vi "Ocean Optics 2000 4000 Acquire Continuous Waveform.vi"() -> ()   [LabVIEW 2024]
doc: "Demonstrates continuous waveform measurement. Spectrum is displayed in a waveform graph."
uses:
  Ocean Optics 2000 4000.lvlib
panel:
  in  "Stop":bool
  out "Spectral Waveform":cluster{dbl[], dbl[]}(graph)
  in  "Enable Strobe (Disabled)":bool
  in  "VISA resource name":refnum<visa-resource-name>
  # "(c) 2009-2016 National Instruments.  ALL RIGHTS RESERVED."
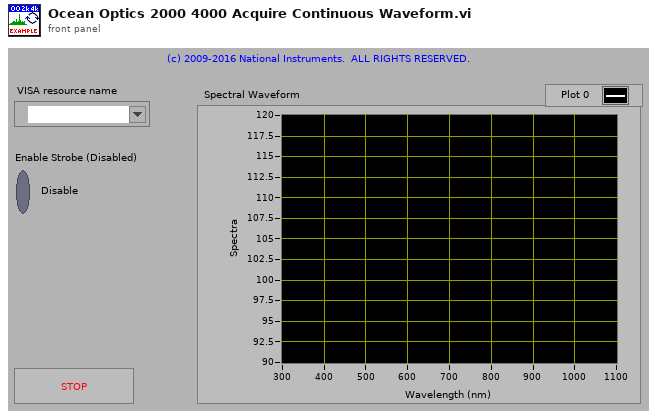
[diagram p1: front panel]
types:
  T1 = cluster{"Wavelength (nm)":dbl[], "Spectrum by Pixel Number":dbl[]}
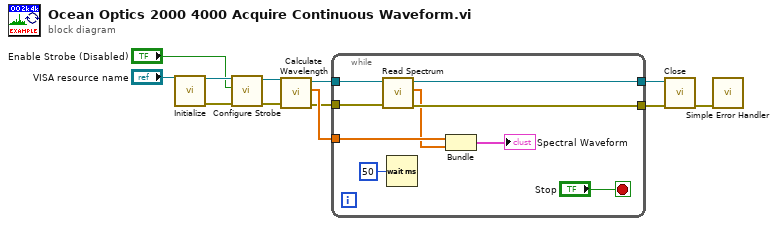
[diagram p0: block diagram]
diagram:
  n1 = call "Initialize.vi"("VISA resource name"="VISA resource name") -> ("error out"=w11:errorcluster, "VISA resource name out"=w12:refnum<visa-resource-name>)  [unwired: 2 in, 7 out]
  n2 = call "Configure Strobe.vi"("error in (no error)"=w11, "Enable Strobe (Disabled)"="Enable Strobe (Disabled)", "VISA resource name"=w12) -> ("error out"=w1:errorcluster, "VISA resource name out"=w2:refnum<visa-resource-name>)  [unwired: 7 out]
  n3 = call "Calculate Wavelength.vi"("error in (no error)"=w1, "VISA resource name"=w2) -> ("error out"=w3:errorcluster, "Wavelength (nm)"=w5:dbl[], "VISA resource name out"=w4:refnum<visa-resource-name>)  [unwired: 1 in, 6 out]
  n4 = while {
    tunnel: [w19] -> w9
    tunnel: [w18] -> w8
    tunnel: w5 -> [w17]
    tunnel: w4 -> [w15]
    tunnel: w3 -> [w14]
    stop <- "Stop" stop-if-true
    n5 = call "Read Spectrum.vi"("error in (no error)"=w14, "VISA resource name"=w15) -> ("error out"=w18:errorcluster, "Spectrum by Pixel Number"=w16:dbl[], "VISA resource name out"=w19:refnum<visa-resource-name>)  [unwired: 6 in, 1 out]
    n6 = Wait (ms)(milliseconds to wait=u32 50 ("millisecond multiple")) -> ()  [unwired: 1 out]
    n7 = Bundle("Wavelength (nm)"=w17, "Spectrum by Pixel Number"=w16) -> (→"Spectral Waveform":T1)  [unwired: 1 out]
  }
  n8 = call "Close.vi"("error in (no error)"=w8, "VISA resource name"=w9) -> ("error out"=w7:errorcluster)  [unwired: 9 out]
  n9 = call <vilib>:"Simple Error Handler.vi"("error in (no error)"=w7) -> ()  [unwired: 1 in, 8 out]
